vi "Wait since.vi"(2 "ms to wait":u32, 3 "Start time":u32) -> (0 "millisecond timer value":u32)   [LabVIEW 2015]
doc: "Much like the LabVIEW \"Wait (ms)\" command, but you also specify a start time that this wait time begins from. You can get this start time from \"Tick Count (ms)\".\n\nAn example: You need to do task A, task B, and task C. You want C to be 100 ms from A, but task B might take a while (and you don't know how long). So do task A, call \"Tick Count (ms)\", do task B, and then call this VI with the start time set as the task A completion time."
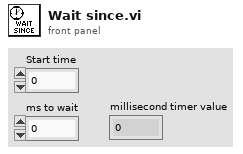
[diagram p1: front panel]
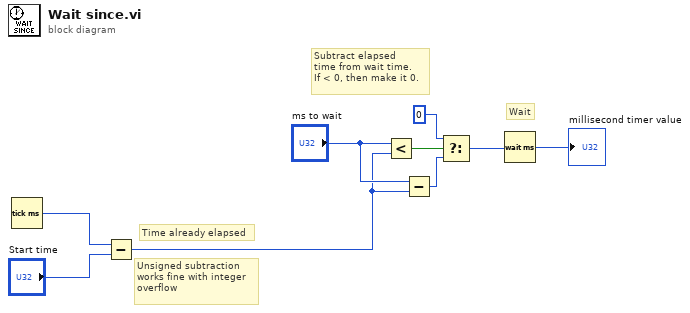
[diagram p0: block diagram]
diagram:
  # "Wait"
  # "Subtract elapsed \ntime from wait time.\nIf < 0, then make it 0."
  # "Unsigned subtraction\nworks fine with integer\noverflow"
  # "Time already elapsed"
  n1 = Tick Count (ms)() -> (millisecond timer value=w9:u32)
  n2 = Subtract(x=w9, y="Start time") -> (x-y=w5:u32)
  n3 = Less?(x="ms to wait", y=w5) -> (x < y?=w7:bool)
  n4 = Subtract(x="ms to wait", y=w5) -> (x-y=w4:u32)
  n5 = Select(t=u32 0, s=w7, f=w4) -> (s? t:f=w2:u32)
  n6 = Wait (ms)(milliseconds to wait=w2) -> (millisecond timer value=→"millisecond timer value":u32)
